vi "GetLoopScript.vi"(8 "ErrorArray":errorcluster[](array[cluster]), 10 "ModuleNames":string[](array[string]), 11 "Test.lvclass":refnum<class "Test.lvclass">) -> (0 "ErrorArray":errorcluster[](array[cluster]), 3 "Test.lvclass":refnum<class "Test.lvclass">)   [LabVIEW 2014, in "Test.lvclass"]
uses:
  Test.lvclass
  Test.lvclass/Test.ctl
  Accessors/Read ErrorSeverity.vi
  Accessors/Read PluginPathArray.vi
  Accessors/Read PluginIndex.vi
  Accessors/Write LoopScript.vi
  <vilib>/Utility/error.llb/Error Cluster From Error Code.vi
  <vilib>/ErrorRing/Error Ring.xnode
  <vilib>/Utility/config.llb/NI_LVConfig.lvlib
  <userlib>/NIST/NISTErrorLib/NISTErrorLib.lvlib
panel:
  # "Usually, the  loop script will be in a single module's .ini file.\nIt is possible that the script will be spread over multiple .ini\nfiles from several modules."
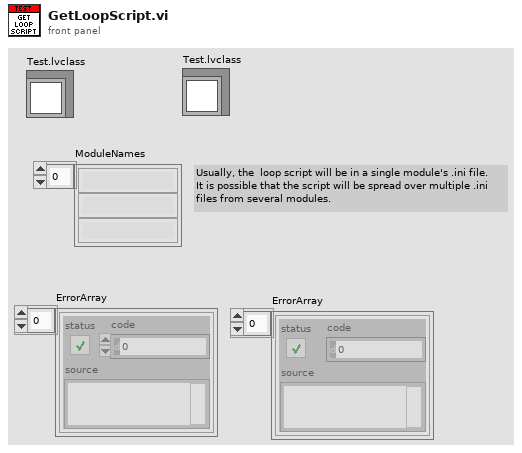
[diagram p1: front panel]
types:
  T1 = typedef "NI_LVConfig.lvlib/Config Data RefNum.ctl" = refnum<k1>
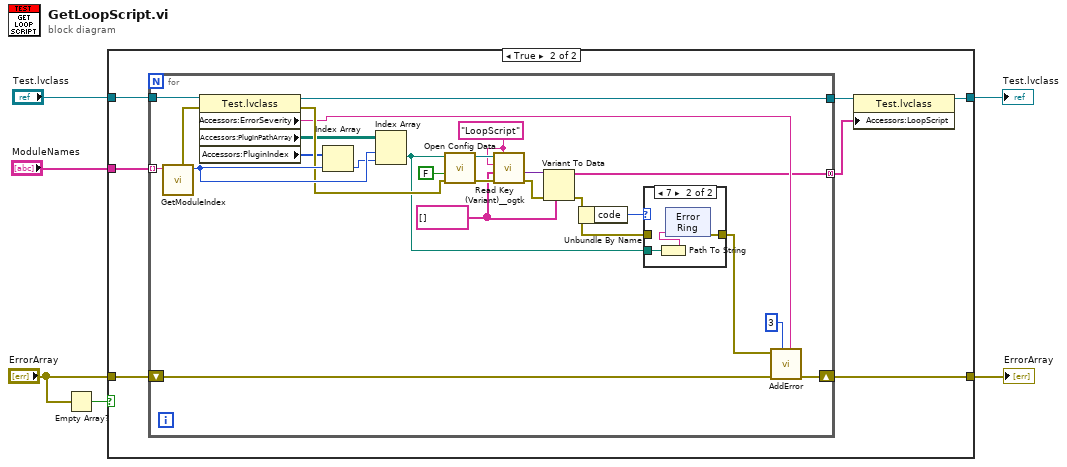
[diagram p0: block diagram]
diagram:
  n1 = Empty Array?(array="ErrorArray") -> (empty?=w6:bool)
  n2 = case shown="True" w6 {
    tunnel: "ErrorArray" -> [w8 w12]
    tunnel: [w8 w11] -> w4
    tunnel: "Test.lvclass" -> [w7 w14]
    tunnel: [w7 w10] -> w2
    tunnel: "ModuleNames" -> [_ w15]
    frame False {
    }
    frame True {
      n3 = for {
        tunnel: w15 -> [w40] mode=indexing
        tunnel: w14 -> [w39]
        tunnel: [w35] -> w13
        shift-right: [w23] -> w11
        shift-left: w12 -> [w34]
        tunnel: [w17] -> w9 mode=concatenating
        w26 = string[] []
        w29 = "LoopScript" ("section")
        n4 = call "GetModuleIndex.vi"("ModuleType"=w40) -> ("ModuleIndex"=w37:i32, "Error"=w38:errorcluster)  [unwired: 9 in]
        n5 = property class="Test.lvclass"(reference=w39, error in=w38) -> (reference out=w35:refnum<class "Test.lvclass">, error out=w32:errorcluster, "Accessors:ErrorSeverity"=w20:string, "Accessors:PluginPathArray"=w21:path[][], "Accessors:PluginIndex"=w22:u32[])
        n6 = Index Array(array=w22, index=w37) -> (element=w36:u32)
        n7 = Index Array(array=w21, index (row)=w37, index (col)=w36) -> (element=w16:path)
        n8 = call <vilib>:"Open Config Data.vi"("error in (no error)"=w32, "create file if necessary (T)"=FALSE, "configuration file path"=w16) -> ("error out"=w31:errorcluster, "refnum"=w30:T1)  [unwired: 6 in, 1 out]
        n9 = call <userlib>:"Read Key (Variant)__ogtk.vi"("section"=w29, "error in (no error)"=w31, "type"=w26, "key (optional)"=w29, "refnum"=w30) -> ("error out"=w28:errorcluster, "key-value"=w27:variant)  [unwired: 3 in, 2 out]
        n10 = Variant To Data(error in=w28, type=w26, Variant=w27) -> (data=w17:string[], error out=w25:errorcluster)
        n11 = Unbundle By Name(w25) -> ("code"=w24:i32)
        n12 = case shown="7" w24 {
          tunnel: w25 -> [w41 _]
          tunnel: [w41 w44] -> w18
          tunnel: w16 -> [_ w43]
          frame 0, Default {
          }
          frame 7 {
            n13 = Path To String(path=w43) -> (string=w42:string)
            n14 = xnode "Error Ring"("parameter 0"=w42) -> ("error out"=w44:errorcluster)
          }
        }
        n15 = call <userlib>:"AddError.vi"("Severity"=w20, "Priority"=u8 3, "ErrorArray"=w34, "error in (no error)"=w18) -> ("ErrorArray"=w23:errorcluster[])  [unwired: 6 in, 1 out]
      }
      n16 = property class="Test.lvclass"(reference=w13, "Accessors:LoopScript"=w9) -> (reference out=w10:refnum<class "Test.lvclass">)  [unwired: 1 in, 1 out]
    }
  }
  "Test.lvclass" <- w2
  "ErrorArray" <- w4
